vi "Time Delay FGV - Saturation.vi"(7 "State":enum16{"Set", "Done?"}(ring), 8 "error in (no error)":errorcluster, 11 "Time to wait (s)":dbl) -> (0 "error out":errorcluster, 2 "Elapsed Time":dbl, 3 "Time's Up!":bool)   [LabVIEW 2017, in "Saturation.lvclass"]
uses:
  Saturation.lvclass
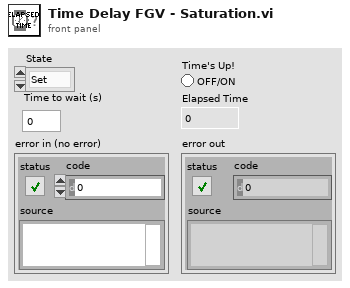
[diagram p1: front panel]
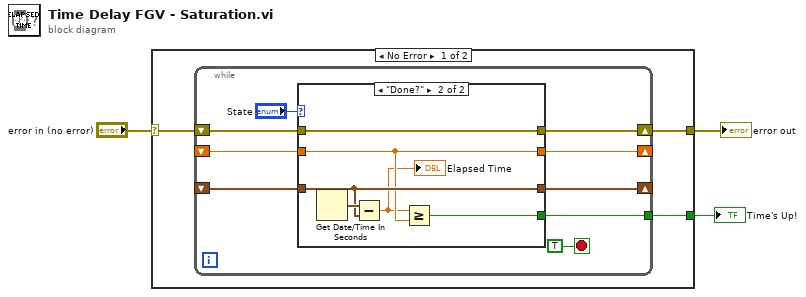
[diagram p0: block diagram]
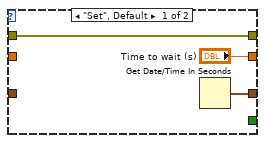
[diagram p2: hidden frame]
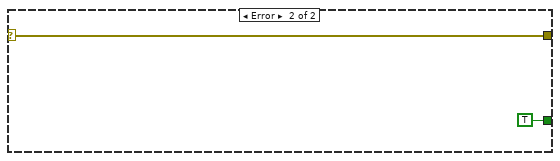
[diagram p3: hidden frame]
diagram:
  n1 = case shown="No Error" "error in (no error)" {
    selector: "error in (no error)" -> [w6 w26]
    tunnel: [w5 w26] -> w2
    tunnel: [w4 TRUE] -> w1
    frame No Error {
      n2 = while {
        shift-right: [w14] -> _
        shift-left: _ -> [w10]
        shift-right: [w12] -> _
        shift-left: _ -> [w11]
        shift-right: [w9] -> w5
        shift-left: w6 -> [w8]
        tunnel: [w7] -> w4
        stop <- TRUE stop-if-true
        n3 = case shown="\"Done?\"" "State" {
          tunnel: ["Time to wait (s)" w21] -> w14
          tunnel: [w17 w23] -> w12
          tunnel: w11 -> [_ w23]
          tunnel: w10 -> [_ w21]
          tunnel: [_ w22] -> w7
          tunnel: [w16 w20] -> w9
          tunnel: w8 -> [w16 w20]
          frame "Set", Default {
            n4 = Get Date/Time In Seconds() -> (seconds since 1Jan1904=w17:timestamp)
          }
          frame "Done?" {
            n5 = Get Date/Time In Seconds() -> (seconds since 1Jan1904=w24:timestamp)
            n6 = Subtract(x=w24, y=w23) -> (x-y=w19:dbl)
            "Elapsed Time" <- w19
            n7 = Greater Or Equal?(x=w19, y=w21) -> (x >= y?=w22:bool)
          }
        }
      }
    }
    frame Error {
    }
  }
  "error out" <- w2
  "Time's Up!" <- w1
